vi "Global 1.vi"() -> ()   [LabVIEW 2020]
panel:
  in  "DUT":i32=1
  out "Voltage Adjusted?":bool
  out "%DiffVoltage":dbl format="%_10g"
  out "VError":dbl format="%_10g"
  out "ReadCurrent":dbl format="%_10g"
  out "ReadVoltage":dbl format="%_10g"
  out "TargetBiasVoltage":dbl format="%_10g"
  out "NewBiasVoltage":dbl format="%_10g"
  out "ArrayCluster2Arrays":cluster{"DUT (x)":dbl[], "DUT (y)":dbl[]}[](array[cluster])
  out "Iteration Leak Comp":i32
  out "Test Comment-GB":string
  out "Device Type-GB":string
  out "Test Type-GB":string
  out "KeystateHP4275AInitSetup":string
  out "Array Size":i32
  out "error out":errorcluster
  out "~~ FINISH ~~":bool
  out "Result - Test Voltages Array":dbl[](array[numeric])
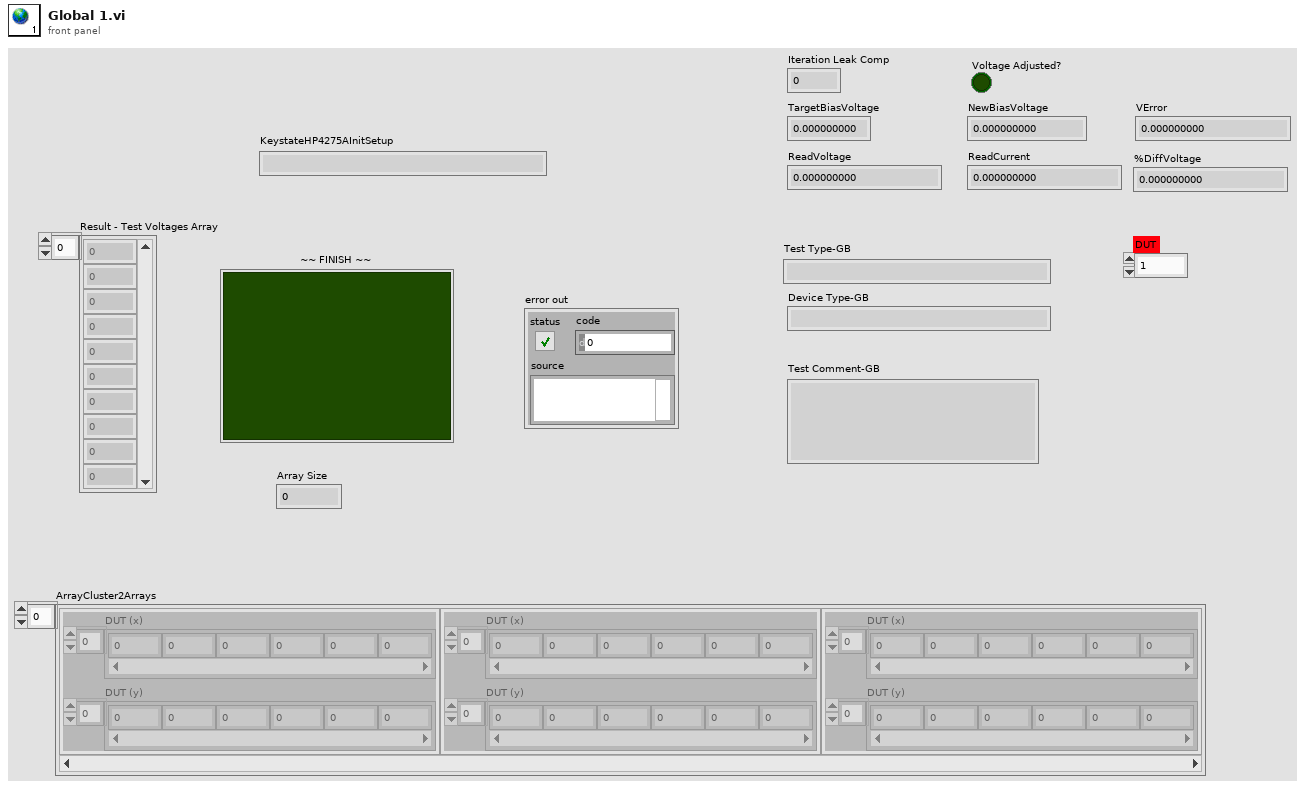
[diagram p1: front panel]
diagram:
